vi "Set DO.vi"(0 "reference in":refnum<class "DO.lvclass">, 1 "Workstation Number":u8, 2 "DO Task Name":string="DO_STAT_1", 3 "DO Module Name":string="DO-Sink-32CH", 5 "error in (no error)":errorcluster, 9 "Physical Channel Numbers":u8[](array[numeric]), 11 "Physical Channel Description":string[](array[string])) -> (14 "reference out":refnum<class "DO.lvclass">, 19 "error out":errorcluster)   [LabVIEW 2017, in "DO.lvclass"]
uses:
  DO.lvclass
  <vilib>/DAQmx/create/channels.llb/DAQmx Create Channel (DO-Digital Output).vi
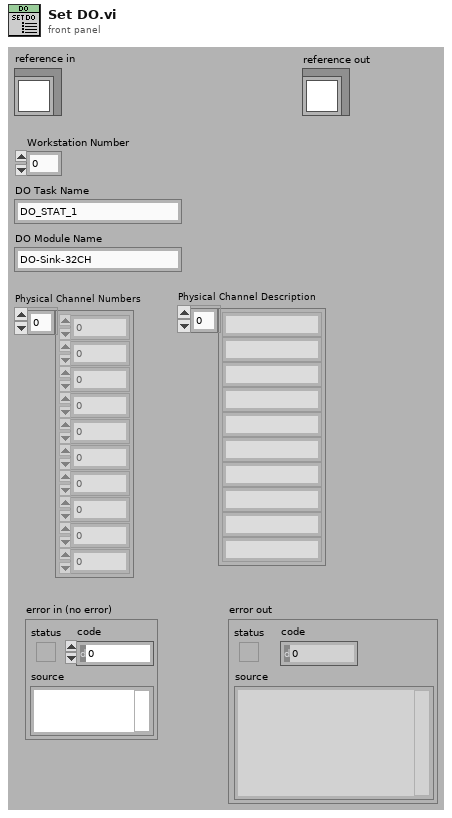
[diagram p1: front panel]
types:
  T1 = typedef "DO.lvclass/ObjectAttributes.ctl" = cluster{"Number of DO Channels in Task":i32, "DO Task":refnum<k21>, "DO Status":bool[], "Physical Channel Description":string[], "Physical Channel Numbers":u8[], "DO Module Name":string, "Workstation Number":u8}
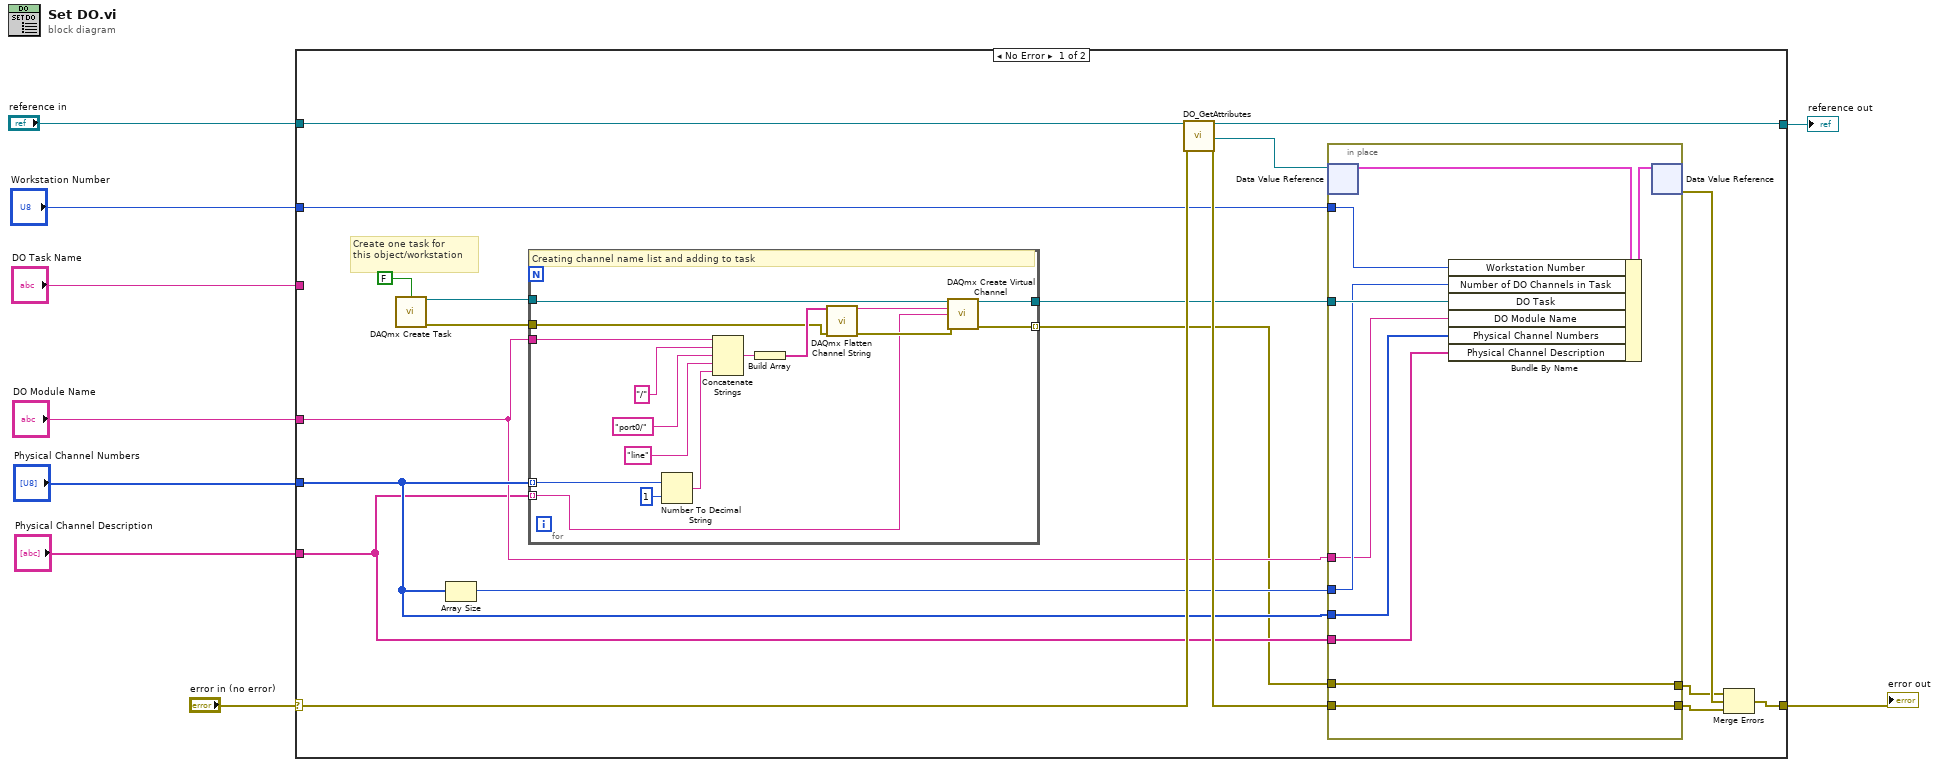
[diagram p0: block diagram]
diagram:
  n1 = case shown="No Error" "error in (no error)" {
    selector: "error in (no error)" -> [w27 w56]
    tunnel: [w24 w56] -> w8
    tunnel: [w25 w55] -> w6
    tunnel: "reference in" -> [w28 w55]
    tunnel: "DO Task Name" -> [_ _]
    tunnel: "Physical Channel Numbers" -> [w18 _]
    tunnel: "DO Module Name" -> [w17 _]
    tunnel: "Physical Channel Description" -> [w16 _]
    tunnel: "Workstation Number" -> [w10 _]
    frame No Error {
      # "Create one task for \nthis object/workstation"
      n2 = call <vilib>:"DAQmx Create Task.vi"("auto cleanup"=FALSE) -> ("task out"=w20:refnum<k21>, "error out"=w15:errorcluster)  [unwired: 13 in]
      n3 = Array Size(array=w18) -> (size(s)=w19:i32)
      n4 = for {
        tunnel: w20 -> [w38]
        tunnel: [w37] -> w14
        tunnel: w18 -> [w34] mode=indexing
        tunnel: w17 -> [w32]
        tunnel: w16 -> [w31] mode=indexing
        tunnel: w15 -> [w30]
        tunnel: [w29] -> w13 mode=indexing
        # "Creating channel name list and adding to task"
        n5 = Number To Decimal String(number=w34, width (-)=i16 1) -> (decimal integer string=w41:string)
        n6 = Concatenate Strings(w32, "/", "port0/", "line", w41) -> (w36:string)
        n7 = Build Array(w36) -> (w35:string[])
        n8 = call <vilib>:"DAQmx Flatten Channel String.vi"("names in"=w35, "error in"=w30) -> ("names out"=w39:string, "error out"=w40:errorcluster)  [unwired: 12 in]
        n9 = call-poly <vilib>:"DAQmx Create Virtual Channel.vi"("task in"=w38, "lines"=w39, "name to assign"=w31, "error in"=w40) -> ("task out"=w37:refnum<k21>, "error out"=w29:errorcluster)  [unwired: 10 in]
      }
      n10 = call "DO_GetAttributes.vi"("reference in"=w28, "error in (no error)"=w27) -> ("reference out"=w25:refnum<class "DO.lvclass">, "DataRef"=w23:refnum<data-value>, "error out"=w22:errorcluster)  [unwired: 14 in, 1 out]
      n11 = in-place {
        in-place-border: w22 -> [w52]
        in-place-border: [w52] -> w21
        in-place-border: w14 -> [w51]
        in-place-border: w19 -> [w50]
        in-place-border: w18 -> [w49]
        in-place-border: w16 -> [w48]
        in-place-border: w17 -> [w47]
        in-place-border: [w46] -> w12
        in-place-border: w13 -> [w46]
        in-place-border: w10 -> [w45]
        n12 = in-place-dvr #1(w23) -> (w53:T1)  [unwired: 1 out]
        n13 = Bundle By Name(cluster=w53, "Workstation Number"=w45, "Number of DO Channels in Task"=w50, "DO Task"=w51, "DO Module Name"=w47, "Physical Channel Numbers"=w49, "Physical Channel Description"=w48) -> (w54:T1)
        n14 = in-place-dvr #1(w54) -> (w26:errorcluster)  [unwired: 1 out]
      }
      n15 = Merge Errors(w12, w26, w21) -> (w24:errorcluster)
    }
    frame Error {
    }
  }
  "error out" <- w8
  "reference out" <- w6
